vi "NF LI56xx dvr sRCL.vi"(8 "error in":errorcluster caption="error in (no error)" {"code" format="%.0x"}, 11 "VISA resource name":refnum<visa-resource-name>) -> (0 "error out":errorcluster {"code" format="%.0x"}, 3 "VISA resource name copy":refnum<visa-resource-name>)   [LabVIEW 2019]
doc: "Restores the settings stored in the specified configuration memory."
panel:
  in  "set memory number":u8 max=9 step=1
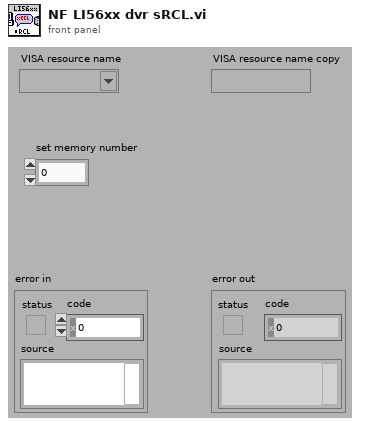
[diagram p1: front panel]
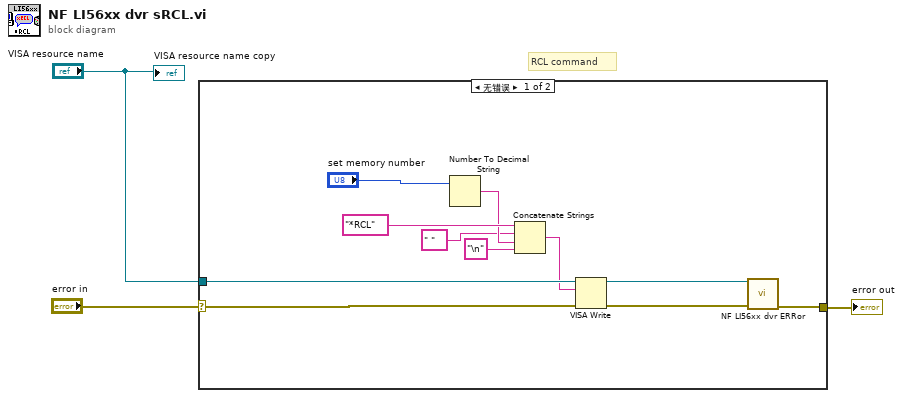
[diagram p0: block diagram]
diagram:
  # "RCL command"
  n1 = case shown="无错误" "error in" {
    selector: "error in" -> [w14 w15]
    tunnel: [w10 w15] -> w3
    tunnel: "VISA resource name" -> [w13 _]
    frame No Error {
      n2 = Number To Decimal String(number="set memory number") -> (decimal integer string=w5:string)  [unwired: 1 in]
      n3 = Concatenate Strings("*RCL" ("•¶Žš—ñ"), " ", w5, "\n" ("Œ`Ž®•¶Žš—ñ")) -> (w9:string)
      n4 = VISA Write(VISA resource name=w13, write buffer=w9, error in (no error)=w14) -> (VISA resource name out=w12:refnum<visa-resource-name>, error out=w11:errorcluster)  [unwired: 1 out]
      n5 = call "NF LI56xx dvr ERRor.vi"("VISA resource name"=w12, "error in (no error)"=w11) -> ("error out"=w10:errorcluster)  [unwired: 10 in, 3 out]
    }
    frame Error {
    }
  }
  "error out" <- w3
  "VISA resource name copy" <- "VISA resource name"
